vi "Clear Class Mutation History.vi"() -> ()   [LabVIEW 2018, in "MVA Framework.lvlib"]
uses:
  MVA Framework.lvlib
  <vilib>/Utility/EditLVLibs/Edit LVLibs.lvlib
panel:
  in  "Application Classes":i32[](listbox)
  in  "Cancel":bool
  in  "Clear":bool
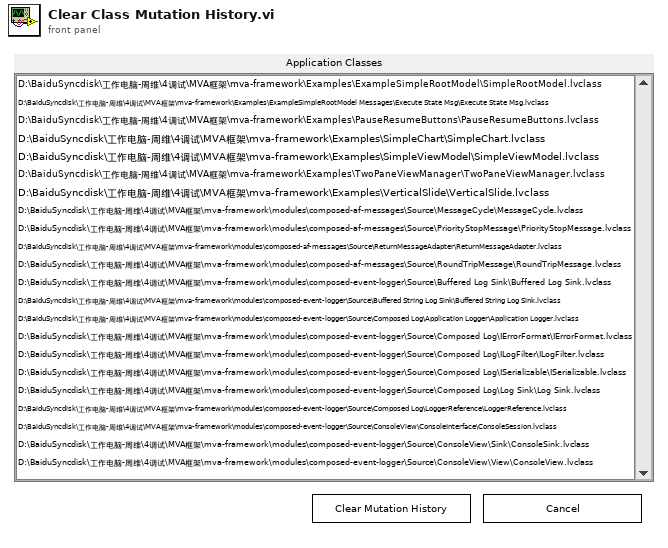
[diagram p1: front panel]
types:
  T1 = typedef "Edit LVLibs.lvlib/Mutation History.ctl" = T2[]
  T2 = typedef "Edit LVLibs.lvlib/Mutation Record.ctl" = cluster{"Library Version":T3, "Old Name Index":u8, "Class Default Data":variant, "Cluster Order Map":u32[], "Parent Name":string, "Parent Path":path, "LabVIEW Version":u32, "User Comments":string, "Mutation Flags":u8, "Parent Old Name Index":u8, "Parent Levels Added":u16, "Parent Levels Removed":u16}
  T3 = typedef "Edit LVLibs.lvlib/LibVersion.ctl" = cluster{"Major":u16, "Minor":u16, "Fix":u16, "Build":u16}
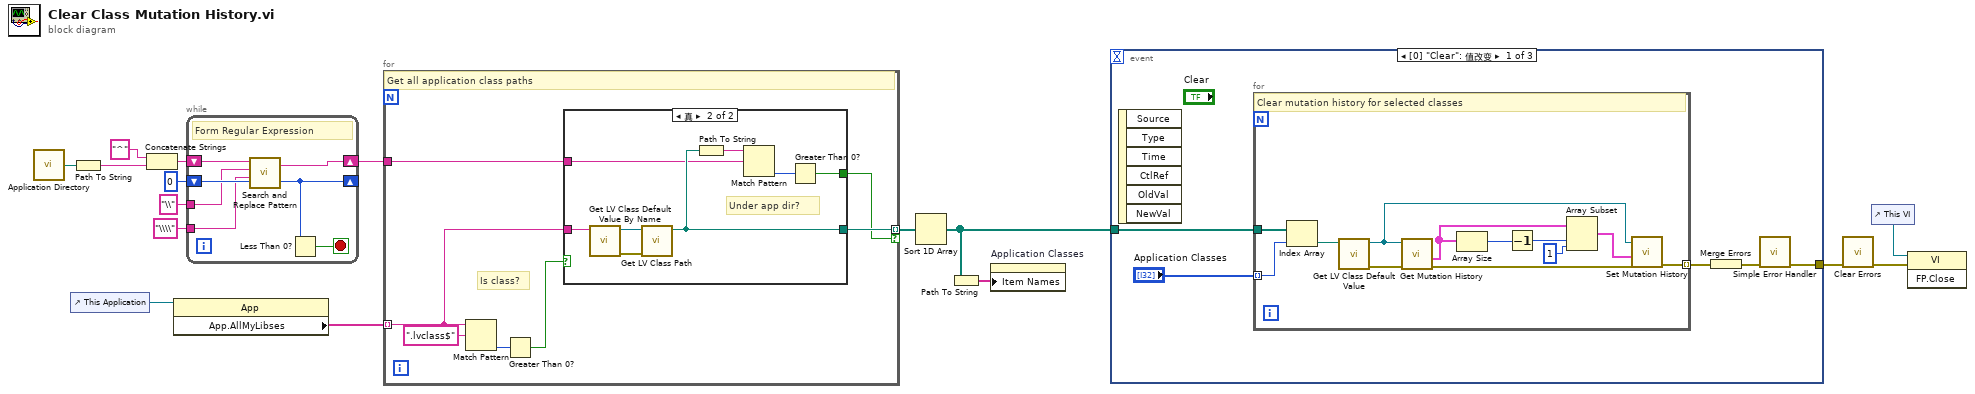
[diagram p0: block diagram]
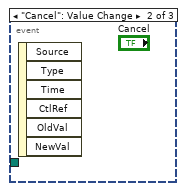
[diagram p2: hidden frame]
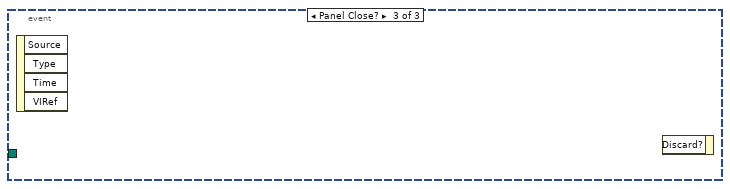
[diagram p3: hidden frame]
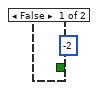
[diagram p4: hidden frame]
diagram:
  n1 = call <vilib>:"Application Directory.vi"() -> ("Application Directory"=w15:path)
  n2 = control-ref of="This Application"() -> (w3:refnum<vi>)
  n3 = Path To String(path=w15) -> (string=w13:string)
  n4 = Concatenate Strings("^" ("string"), w13) -> (w11:string)
  n5 = property class="App"(reference=w3) -> ("App.AllMyLibses"=w16:string[])  [unwired: 1 in, 2 out]
  n6 = while {
    shift-right: [w23] -> w12
    shift-left: w11 -> [w22]
    shift-right: [w20] -> _
    shift-left: 0 ("offset past match") -> [w21]
    tunnel: "\\\\" ("replace string (\"\")") -> [w19]
    tunnel: "\\" ("regular expression (\"\")") -> [w18]
    stop <- w17 stop-if-true
    # "Form Regular Expression"
    n7 = call <vilib>:"Search and Replace Pattern.vi"("string"=w22, "regular expression (\"\")"=w18, "replace string (\"\")"=w19, "offset (0)"=w21) -> ("result string"=w23:string, "offset past match"=w20:i32)  [unwired: 1 in]
    n8 = Less Than 0?(x=w20) -> (x < 0?=w17:bool)
  }
  n9 = for {
    tunnel: w16 -> [w28] mode=indexing
    tunnel: [w27] -> w7 mode=indexing if=w24
    tunnel: w12 -> [w25]
    # "Is class?"
    # "Get all application class paths"
    n10 = Match Pattern(string=w28, regular expression=".lvclass$") -> (offset past match=w29:i32)  [unwired: 1 in, 3 out]
    n11 = Greater Than 0?(x=w29) -> (x > 0?=w26:bool)
    n12 = case shown="真" w26 {
      tunnel: w28 -> [_ w36]
      tunnel: [_ w35] -> w27
      tunnel: w25 -> [_ w32]
      tunnel: [_ w34] -> w24
      frame False {
        (unwired) -2 ("offset past match")
      }
      frame True {
        # "Under app dir?"
        n13 = call <vilib>:"Get LV Class Default Value By Name.vi"("class name"=w36) -> ("error out"=w37:errorcluster, "object"=w38:refnum<class>)  [unwired: 9 in]
        n14 = call <vilib>:"Get LV Class Path.vi"("error in (no error)"=w37, "object"=w38) -> ("class path"=w35:path)  [unwired: 8 in, 1 out]
        n15 = Path To String(path=w35) -> (string=w33:string)
        n16 = Match Pattern(string=w33, regular expression=w32) -> (offset past match=w31:i32)  [unwired: 1 in, 3 out]
        n17 = Greater Than 0?(x=w31) -> (x > 0?=w34:bool)
      }
    }
  }
  n18 = Sort 1D Array(array=w7) -> (sorted array=w1:path[])
  n19 = Path To String(path=w1) -> (string=w6:string[])
  n20 = property on="Application Classes" class="LstBox (严格)"("Item Names"=w6) -> ()  [unwired: 2 in, 2 out]
  n21 = event shown="[0] \"Clear\": 值改变" {
    selector: _ -> [_ _ _]
    dyn-events: _ -> [_ _ _]
    timeout: _ -> [_ _ _]
    tunnel: w1 -> [w43 _ _]
    tunnel: [w39 _ _] -> w5
    event "Clear": Value Change {
      n22 = event-data() -> ()  [unwired: 1 in, 6 out]
      n23 = for {
        tunnel: w43 -> [w46]
        tunnel: [w47] -> w42 mode=indexing
        tunnel: "Application Classes" -> [w44] mode=indexing
        # "Clear mutation history for selected classes"
        n24 = Index Array(array=w46, index=w44) -> (element=w45:path)
        n25 = call <vilib>:"Get LV Class Default Value.vi"("class path"=w45) -> ("error out"=w55:errorcluster, "object"=w48:refnum<class>)  [unwired: 9 in]
        n26 = call <vilib>:"Get Mutation History.vi"("error in"=w55, "Input object"=w48) -> ("error out"=w49:errorcluster, "Mutation History"=w53:T1)  [unwired: 6 in]
        n27 = Array Size(array=w53) -> (size(s)=w54:i32)
        n28 = Decrement(x=w54) -> (x-1=w52:i32)
        n29 = Array Subset(array=w53, index=w52, length=1) -> (w50:T1)
        n30 = call <vilib>:"Set Mutation History.vi"("error in"=w49, "Mutation History"=w50, "Input object"=w48) -> ("error out"=w47:errorcluster)  [unwired: 8 in]
      }
      n31 = Merge Errors(w42) -> (w41:errorcluster)
      n32 = call <vilib>:"Simple Error Handler.vi"("error in (no error)"=w41) -> ("error out"=w39:errorcluster)  [unwired: 4 in, 4 out]
    }
    event "Cancel": Value Change {
      n33 = event-data() -> ()  [unwired: 1 in, 6 out]
    }
    event Panel Close? {
      n34 = event-data() -> ()  [unwired: 1 in, 4 out]
      n35 = event-data() -> ()  [unwired: 2 in, 1 out]
    }
  }
  n36 = call <vilib>:"Clear Errors.vi"("error in (no error)"=w5) -> ("error out"=w4:errorcluster)  [unwired: 5 in, 1 out]
  n37 = control-ref of="This VI"() -> (w2:refnum<vi>)
  n38 = invoke class="VI" method="FP.Close"(reference=w2, error in=w4) -> ()  [unwired: 1 in, 3 out]
